vi "Modify Swerve.vi"(0 "Original":T1[](array[typedef]), 1 "mode":u32(ring) items=["SWERVE_DEFAULT"], 2 "wheelbase_depth":dbl, 3 "wheelbase_width":dbl, 5 "error in":errorcluster) -> (14 "Original":T1[](array[typedef]), 15 "front_left out":T1[](array[typedef]), 16 "front_right out":T1[](array[typedef]), 17 "back_left out":T1[](array[typedef]), 18 "back_right out":T1[](array[typedef]), 19 "error out":errorcluster)   [LabVIEW 2017, in "Pathfinder.lvlib"]
doc: "CAPI void pathfinder_modify_swerve(Segment *original, int length, Segment *front_left, Segment *front_right,\n Segment *back_left, Segment *back_right, double wheelbase_width, double wheelbase_depth, SWERVE_MODE mode);"
uses:
  Pathfinder.lvlib
  Segment.ctl
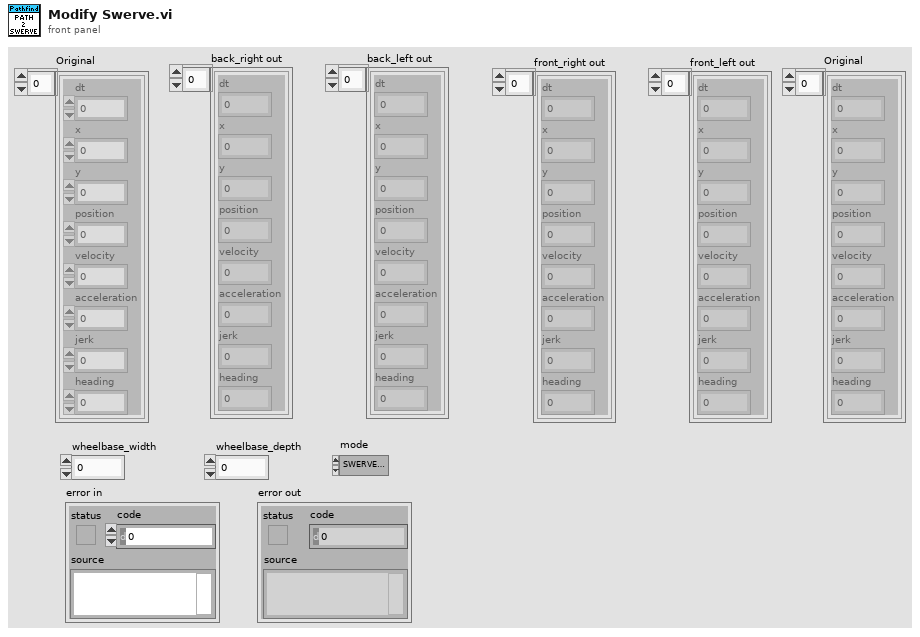
[diagram p1: front panel]
types:
  T1 = typedef "Pathfinder.lvlib/Segment.ctl" = cluster{"dt":dbl, "x":dbl, "y":dbl, "position":dbl, "velocity":dbl, "acceleration":dbl, "jerk":dbl, "heading":dbl}
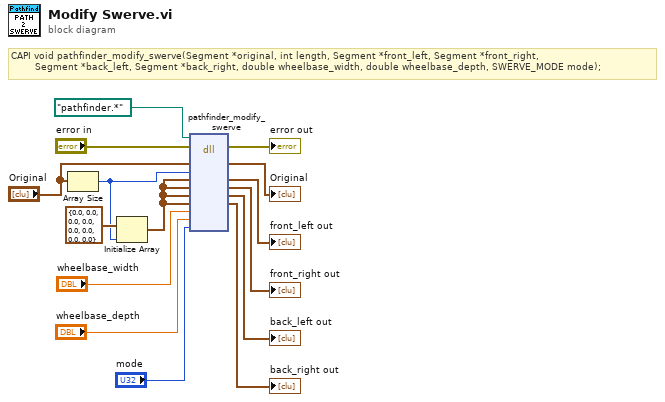
[diagram p0: block diagram]
diagram:
  # "CAPI void pathfinder_modify_swerve(Segment *original, int length, Segment *front_left, Segment *front_right,\n        Segment *back_left, Segment *back_right, double wheelbase_width, double wheelbase_depth, SWERVE_MODE mode);"
  n1 = Array Size(array="Original") -> (size(s)=w3:i32)
  n2 = Initialize Array(T1 {"dt"=0.0, "x"=0.0, "y"=0.0, "position"=0.0, "velocity"=0.0, "acceleration"=0.0, "jerk"=0.0, "heading"=0.0} ("segment"), w3) -> (w8:T1[])
  n3 = dll-call lib="?" fn="pathfinder_modify_swerve"(path in=path "pathfinder.*", error in="error in", "original"="Original", "length"=w3, "front_left"=w8, "front_right"=w8, "back_left"=w8, "back_right"=w8, "wheelbase_width"="wheelbase_width", "wheelbase_depth"="wheelbase_depth", "mode"="mode") -> (error out=→"error out":errorcluster, "original"=→"Original":T1[], "front_left"=→"front_left out":T1[], "front_right"=→"front_right out":T1[], "back_left"=→"back_left out":T1[], "back_right"=→"back_right out":T1[])  [unwired: 6 in, 1 out]
